vi "Memory.Pointer.Internal.Dispose.vi"(8 "error in (no error)":errorcluster, 11 "pointer":refnum<class "Memory.Pointer.Internal.lvclass">) -> (0 "error out":errorcluster)   [LabVIEW 2016, in "Memory Manager.lvlib" / "Memory.Pointer.Internal.lvclass"]
doc: "Disposes of the provided <b>pointer</b> and deallocates the associated memory."
uses:
  Memory.Pointer.Internal.lvclass
  C:/Users/Ryan/Documents/Git/Sourcetree/LabVIEW-Memory-Manager/Source/Library/Classes/Pointer/Memory.Pointer.lvclass
  Pointer/Memory.Pointer.lvclass/Memory.Pointer.ctl
  Pointer/Methods/Memory.Pointer.Errors.Zone.vi
  Pointer/Methods/Memory.Pointer.Errors.Null Pointer.vi
  Pointer/Methods/Memory.Pointer.Errors.Create Error.vi
  Submodules/Static Error Handling/Source/Library/VIs/Static Error Handling.Error Cluster Constant.vi
  Submodules/Static Error Handling/Source/Library/VIs/Static Error Handling.Error Cluster Constant (256B).vi
  Submodules/Static Error Handling/Source/Library/VIs/Static Error Handling.Parameters.Status.Set.vi
  Submodules/Static Error Handling/Source/Library/VIs/Static Error Handling.Parameters.Code.Set.vi
  Submodules/Static Error Handling/Source/Library/VIs/Static Error Handling.Parameters.VI Source.Set.vi
  Constants/Memory.Constants.vi
  Constants/Memory.Constants.Library Name.vi
  Pointer/Methods/Memory.Pointer.Errors.Get Info.vi
  Submodules/Static Error Handling/Source/Library/VIs/Static Error Handling.Source Buffer.Write.String.vi
  Pointer/Memory.Pointer.lvclass
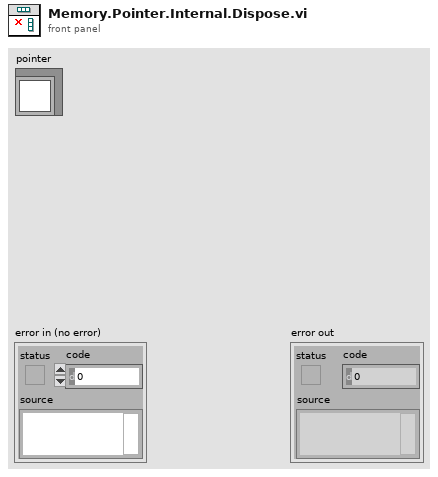
[diagram p1: front panel]
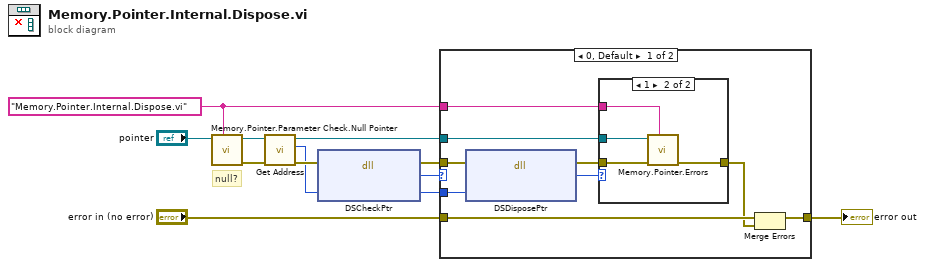
[diagram p0: block diagram]
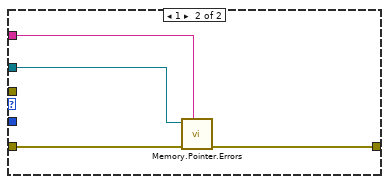
[diagram p3: hidden frame]
diagram:
  w1 = "Memory.Pointer.Internal.Dispose.vi" ("source vi name")
  # "null?"
  n1 = call "Memory.Pointer.Parameter Check.Null Pointer.vi"("source vi name"=w1, "Pointer in"="pointer") -> ("error out"=w4:errorcluster, "Pointer out"=w6:refnum<class "Memory.Pointer.Internal.lvclass">)  [unwired: 8 in]
  n2 = call "Get Address.vi"("error in (no error)"=w4, "Pointer in"=w6) -> ("error out"=w5:errorcluster, "address"=w3:u64, "Pointer out"=w10:refnum<class "Memory.Pointer.Internal.lvclass">)  [unwired: 7 in]
  n3 = dll-call lib="LabVIEW" fn="DSCheckPtr"(error in=w5, "pointer"=w3) -> (error out=w11:errorcluster, "return"=w9:i32, "pointer"=w8:u64)  [unwired: 2 in, 1 out]
  n4 = case shown="0, Default" w9 {
    tunnel: [w21 w29] -> w12
    tunnel: "error in (no error)" -> [w20 w30]
    tunnel: w1 -> [w19 w28]
    tunnel: w10 -> [w15 w27]
    tunnel: w11 -> [w14 _]
    tunnel: w8 -> [w13 _]
    frame 0, Default {
      n5 = dll-call lib="LabVIEW" fn="DSDisposePtr"(error in=w14, "pointer"=w13) -> (error out=w18:errorcluster, "return"=w17:i32)  [unwired: 3 in, 1 out]
      n6 = case shown="1" w17 {
        tunnel: w18 -> [w22 w26]
        tunnel: [w22 w25] -> w16
        tunnel: w15 -> [_ w24]
        tunnel: w19 -> [_ w23]
        frame 0, Default {
        }
        frame 1 {
          n7 = call-poly "Memory.Pointer.Errors.vi"("source vi name"=w23, "error in (no error)"=w26, "pointer in"=w24) -> ("error out"=w25:errorcluster)  [unwired: 7 in, 1 out]
        }
      }
      n8 = Merge Errors(w20, w16) -> (w21:errorcluster)
    }
    frame 1 {
      n9 = call-poly "Memory.Pointer.Errors.vi"("source vi name"=w28, "error in (no error)"=w30, "pointer in"=w27) -> ("error out"=w29:errorcluster)  [unwired: 7 in, 1 out]
    }
  }
  "error out" <- w12
